vi "Get Error.vi"(3 "Report (T)":bool=TRUE, 4 "Error Additional Information":string, 5 "Error":T1) -> (0 "source":string, 1 "code":i32, 2 "Error out":errorcluster)   [LabVIEW 2023, in "Iterator Actor.lvlib" / "Abstract Iterator Actor.lvclass"]
doc: "Generates a specific Iterator error depending on the input value. Error codes are summarized in the Documentation for the project."
uses:
  Abstract Iterator Actor.lvclass
  Iterator Errors.ctl
  <vilib>/Utility/error.llb/Trim Whitespace One-Sided.vi
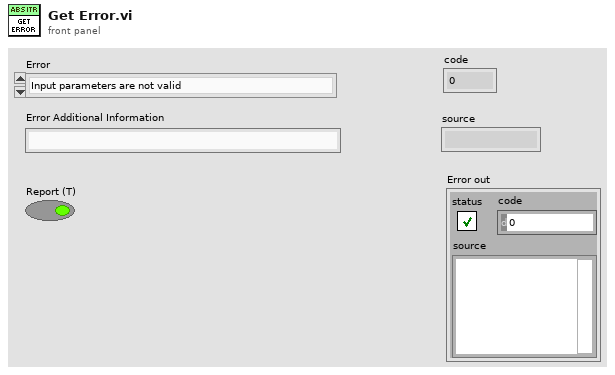
[diagram p1: front panel]
types:
  T1 = typedef "Iterator Actor.lvlib/Abstract Iterator Actor.lvclass/Iterator Errors.ctl" = enum16{"Input parameters are not valid", "Preparation call timed out", "Iteration call timed out", "Conclusion call timed out"}
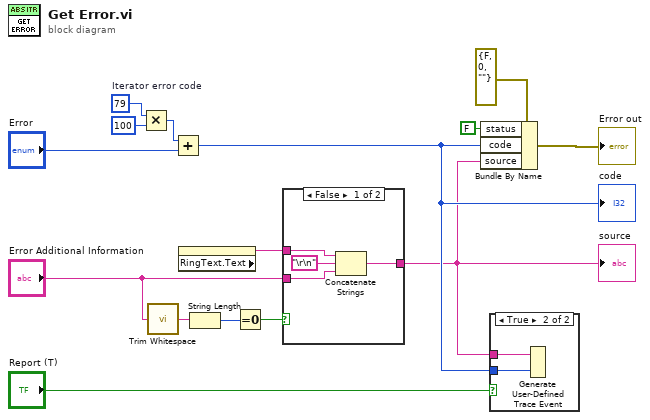
[diagram p0: block diagram]
diagram:
  w12 = 79  # Iterator error code
  n1 = Multiply(x=w12, y=100 ("code")) -> (x*y=w11:i32)
  n2 = call <vilib>:"Trim Whitespace.vi"("string"="Error Additional Information") -> ("trimmed string"=w5:string)  [unwired: 1 in]
  n3 = Add(x=w11, y="Error") -> (x+y=w2:i32)
  "code" <- w2
  n4 = property on="Error" class="Enum (strict)"() -> ("RingText.Text"=w3:string)  [unwired: 2 in, 2 out]
  n5 = String Length(string=w5) -> (length=w8:i32)
  n6 = Equal To 0?(x=w8) -> (x = 0?=w6:bool)
  n7 = case shown="False" w6 {
    tunnel: w3 -> [w18 w20]
    tunnel: [w17 w20] -> w1
    tunnel: "Error Additional Information" -> [w16 _]
    frame False {
      n8 = Concatenate Strings(w18, "\r\n", w16) -> (w17:string)
    }
    frame True {
    }
  }
  "source" <- w1
  n9 = Bundle By Name(cluster=errorcluster {"status"=FALSE, "code"=0, "source"=""} ("error constant"), "status"=FALSE, "code"=w2, "source"=w1) -> (→"Error out":errorcluster)
  n10 = case shown="True" "Report (T)" {
    tunnel: w1 -> [_ w22]
    tunnel: w2 -> [_ w21]
    frame False {
    }
    frame True {
      n11 = Generate User-Defined Trace Event(1:w21, 2:w22) -> ()
    }
  }
